vi "DrawAxes.vi"(3 "Colors":T2={"X Color"=16716800, "Y Color"=6618880, "Z Color"=7451135}, 4 "Axes":T1=[[1.0, 0.0, 0.0, 0.0], [0.0, 1.0, 0.0, 0.0], [0.0, 0.0, 1.0, 0.0], [0.0, 0.0, 0.0, 1.0]], 5 "Stage in":refnum<vi>) -> (2 "Stage out":refnum<vi>)   [LabVIEW 2024]
uses:
  <vilib>/Analysis/Matrix/Datatypes/RealMatrix.ctl
  <vilib>/picture/3D Picture Control/NI_3D Picture Control.lvlib
  <vilib>/Analysis/Matrix/NI_Matrix.lvlib
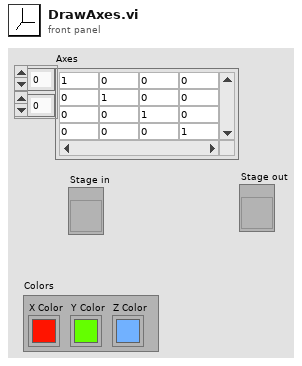
[diagram p1: front panel]
types:
  T1 = typedef "NI_Matrix.lvlib/RealMatrix.ctl" = dbl[][]
  T2 = cluster{"X Color":u32, "Y Color":u32, "Z Color":u32}
  T3 = cluster{"Axes[0]":dbl, "Axes[1]":dbl, "Axes[2]":dbl}
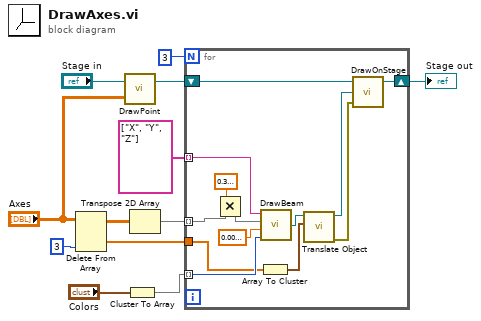
[diagram p0: block diagram]
diagram:
  n1 = Delete From Array(array="Axes", index (col)=3 ("disabled index (col)")) -> (deleted portion=w1:dbl[], array with subset deleted=w6:T1)  [unwired: 2 in]
  n2 = call <userlib>:"DrawPoint.vi"("Start"="Axes", "Stage in"="Stage in") -> ("Stage out"=w8:refnum<vi>)  [unwired: 1 in]
  n3 = Cluster To Array(cluster="Colors") -> (array=w11:u32[])
  n4 = Transpose 2D Array(2D array=w6) -> (transposed array=w3:T1)
  n5 = for {
    N: 3 -> [_]
    tunnel: w3 -> [w14] mode=indexing
    tunnel: w1 -> [w18]
    shift-right: [w16] -> w5
    shift-left: w8 -> [w25]
    tunnel: w11 -> [w23] mode=indexing
    tunnel: string[] ["X", "Y", "Z"] -> [w24] mode=indexing
    n6 = Multiply(x=sgl 0.3 ("Beam radius"), y=w14) -> (x*y=w13:dbl[])
    n7 = Array To Cluster(array=w18) -> (cluster=w19:T3)
    n8 = call <userlib>:"DrawBeam.vi"("Color"=w23, "Beam radius"=sgl 0.01, "Point"=w13, "Name"=w24) -> ("Beam"=w21:refnum<vi>)  [unwired: 2 in]
    n9 = call <vilib>:"Translate Object.vi"("Translation"=w19, "Scene.Object In"=w21) -> ("error out"=w22:errorcluster, "Scene.Object Out"=w20:refnum<vi>)  [unwired: 8 in]
    n10 = call <userlib>:"DrawOnStage.vi"("error in"=w22, "object in"=w20, "Stage in"=w25) -> ("Stage out"=w16:refnum<vi>)  [unwired: 2 out]
  }
  "Stage out" <- w5
